vi "strings to line.vi"(11 "strings":string[](array[string])) -> (3 "line":T1)   [LabVIEW 2013, in "EthernetIP editor node.lvclass"]
uses:
  EthernetIP editor node.lvclass
  table line.ctl
  <vilib>/NI/TBM Modules/Ethernet IP/channel/EthernetIP Channel.lvclass
  <vilib>/NI/Tag Bus/tag/Data Type.ctl
  <vilib>/NI/TBM Modules/Ethernet IP/configuration/assembly type.ctl
  <vilib>/NI/Tag Bus/tag/tag descriptor.lvclass
  <vilib>/NI/TBM Modules/Ethernet IP/configuration/EthernetIP configuration.lvclass
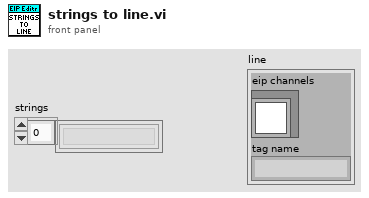
[diagram p1: front panel]
types:
  T1 = typedef "EthernetIP editor node.lvclass/table line.ctl" = cluster{"eip channels":refnum<class "EthernetIP Channel.lvclass">, "tag name":string}
  T2 = typedef "EthernetIP configuration.lvclass/assembly type.ctl" = enum32{"Producing", "Consuming"}
  T3 = typedef "tag bus.lvlib/tag descriptor.lvclass/Data Type.ctl" = enum16{"Double", "Single", "I64", "I32", "I16", "I8", "U64", "U32", "U16", "U8", "Boolean", "String", "Array of Double", "Array of Single", "Array of I64", "Array of I32", "Array of I16", "Array of I8", "Array of U64", "Array of U32", "Array of U16", "Array of U8", "Array of Boolean", "Array of String"}
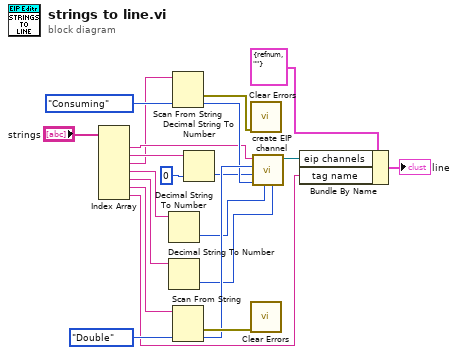
[diagram p0: block diagram]
diagram:
  n1 = Index Array(array="strings") -> (element #1=w11:string, element #2=w10:string, element #3=w7:string, element #4=w4:string, element #5=w3:string, element #6=w2:string, element #7=w1:string)  [unwired: 7 in]
  n2 = Decimal String To Number(string=w4) -> (number=w6:i32)  [unwired: 2 in, 1 out]
  n3 = Decimal String To Number(string=w3) -> (number=w5:i32)  [unwired: 2 in, 1 out]
  n4 = Scan From String(input string=w7, default 1=assembly_type."Consuming" ("Type")) -> (error out=w16:errorcluster, output 1=w12:T2)  [unwired: 3 in, 2 out]
  n5 = Scan From String(input string=w2, default 1=Data_Type."Double" ("data type")) -> (error out=w18:errorcluster, output 1=w13:T3)  [unwired: 3 in, 2 out]
  n6 = Decimal String To Number(string=w10, default (0L)=u32 0 ("Instance ID")) -> (number=w8:u32)  [unwired: 1 in, 1 out]
  n7 = call <vilib>:"Clear Errors.vi"("error in (no error)"=w16) -> ()  [unwired: 6 in, 1 out]
  n8 = call <vilib>:"Clear Errors.vi"("error in (no error)"=w18) -> ()  [unwired: 6 in, 1 out]
  n9 = call <vilib>:"create EIP channel.vi"("subindex"=w5, "byte index"=w6, "Type"=w12, "Instance ID"=w8, "data type"=w13, "name"=w11) -> ("EthernetIP Channel out"=w14:refnum<class "EthernetIP Channel.lvclass">)  [unwired: 5 in]
  n10 = Bundle By Name(cluster=T1 {"eip channels"=refnum, "tag name"=""} ("line"), "eip channels"=w14, "tag name"=w1) -> (→"line":T1)
